vi "MoAgSy_AgentBase_GPG_keyring.vi"(0 "HGF_Agent in":refnum<class "MoAgSy_AgentBase.lvclass">, 2 "key":string, 5 "error in (no error)":errorcluster, 8 "Enum":T1(ring)) -> (14 "HGF_Agent out":refnum<class "MoAgSy_AgentBase.lvclass">, 16 "pub keys":string[](array[string]), 17 "Key":string, 19 "error out":errorcluster)   [LabVIEW 2009, in "MoAgSy_Base.lvlib" / "MoAgSy_AgentBase.lvclass"]
uses:
  MoAgSy_AgentBase.lvclass
  MoAgSy_AgentBase.lvclass/MoAgSy_AgentBase.ctl
  MoAgSy_GPG/MoAgSy_GPG.lvclass
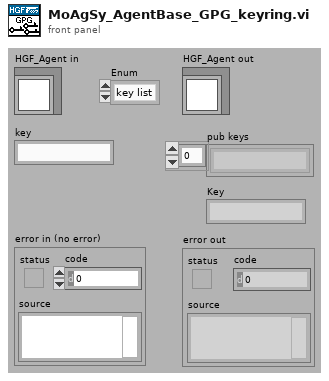
[diagram p1: front panel]
types:
  T1 = enum16{"key list", "pub key", "delete key", "add key", "local sign key"}
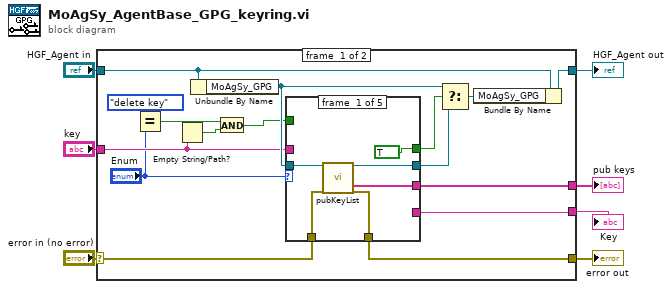
[diagram p0: block diagram]
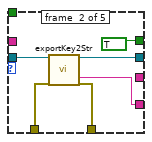
[diagram p2: hidden frame]
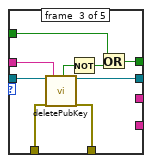
[diagram p3: hidden frame]
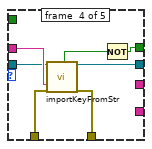
[diagram p4: hidden frame]
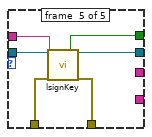
[diagram p5: hidden frame]
diagram:
  n1 = case shown="No Error" "error in (no error)" {
    selector: "error in (no error)" -> [w13 w59]
    tunnel: [w17 w59] -> w6
    tunnel: [w22 w58] -> w4
    tunnel: "HGF_Agent in" -> [w23 w58]
    tunnel: [w16 _] -> w3
    tunnel: [w15 _] -> w2
    tunnel: "key" -> [w14 _]
    frame #0 {
      n2 = Equal?(x=T1."delete key" ("y"), y="Enum") -> (x = y?=w10:bool)
      n3 = Empty String/Path?(string/path=w14) -> (empty?=w9:bool)
      n4 = Unbundle By Name(w23) -> ("MoAgSy_GPG"=w21:refnum<class "MoAgSy_GPG.lvclass">)
      n5 = And(x=w10, y=w9) -> (x .and. y?=w8:bool)
      n6 = case shown="\"local sign key\"" "Enum" {
        tunnel: w21 -> [w29 w35 w44 w48 w57]
        tunnel: [TRUE TRUE w37 w45 w52] -> w19
        tunnel: [w27 w34 w43 w47 w56] -> w18
        tunnel: w13 -> [w26 w32 w42 w50 w54]
        tunnel: [w25 w31 w41 w49 w53] -> w17
        tunnel: [w24 _ _ _ _] -> w16
        tunnel: [_ w30 _ _ _] -> w15
        tunnel: w14 -> [_ _ w40 w51 w55]
        tunnel: w8 -> [_ _ w36 _ _]
        frame #0 {
          n7 = call-dynamic "pubKeyList.vi"("HGF_GPG in"=w29, "error in (no error)"=w26) -> ("HGF_GPG out"=w27:refnum<class "MoAgSy_GPG.lvclass">, "pub keys"=w24:string[], "error out"=w25:errorcluster)  [unwired: 4 in, 11 out]
        }
        frame #1 {
          n8 = call-dynamic "exportKey2Str.vi"("HGF_GPG in"=w35, "error in (no error)"=w32) -> ("HGF_GPG out"=w34:refnum<class "MoAgSy_GPG.lvclass">, "Key"=w30:string, "error out"=w31:errorcluster)  [unwired: 6 in, 9 out]
        }
        frame #2 {
          n9 = call-dynamic "deletePubKey.vi"("HGF_GPG in"=w44, "error in (no error)"=w42, "key-id"=w40) -> ("success"=w39:bool, "HGF_GPG out"=w43:refnum<class "MoAgSy_GPG.lvclass">, "error out"=w41:errorcluster)  [unwired: 4 in, 10 out]
          n10 = Not(x=w39) -> (.not. x?=w38:bool)
          n11 = Or(x=w36, y=w38) -> (x .or. y?=w37:bool)
        }
        frame #3 {
          n12 = call-dynamic "importKeyFromStr.vi"("HGF_GPG in"=w48, "key"=w51, "error in (no error)"=w50) -> ("success"=w46:bool, "HGF_GPG out"=w47:refnum<class "MoAgSy_GPG.lvclass">, "error out"=w49:errorcluster)  [unwired: 4 in, 10 out]
          n13 = Not(x=w46) -> (.not. x?=w45:bool)
        }
        frame #4 {
          n14 = call-dynamic "lsignKey.vi"("MoAgSy_GPG"=w57, "id2sign"=w55, "error in (no error)"=w54) -> ("data error?"=w52:bool, "dup MoAgSy_GPG"=w56:refnum<class "MoAgSy_GPG.lvclass">, "error out"=w53:errorcluster)  [unwired: 6 in, 8 out]
        }
      }
      n15 = Select(t=w21, s=w19, f=w18) -> (s? t:f=w20:refnum<class "MoAgSy_GPG.lvclass">)
      n16 = Bundle By Name(cluster=w23, "MoAgSy_GPG"=w20) -> (w22:refnum<class "MoAgSy_AgentBase.lvclass">)
    }
    frame #1 {
    }
  }
  "error out" <- w6
  "HGF_Agent out" <- w4
  "pub keys" <- w3
  "Key" <- w2
